vi "getNodeName.vi"(8 "error in (no error)":errorcluster, 11 "NativeXML in":refnum<class "NativeXML.lvclass">) -> (0 "error out":errorcluster, 2 "name":string, 3 "NativeXML out":refnum<class "NativeXML.lvclass">)   [LabVIEW 2011, in "Tools.lvlib" / "xml.lvlib" / "NativeXML.lvclass"]
uses:
  NativeXML.lvclass
  NativeXML.lvclass/NativeXML.ctl
  Program Files/National Instruments/LabVIEW 2011/resource/objmgr/DOMUserDefRef.rc
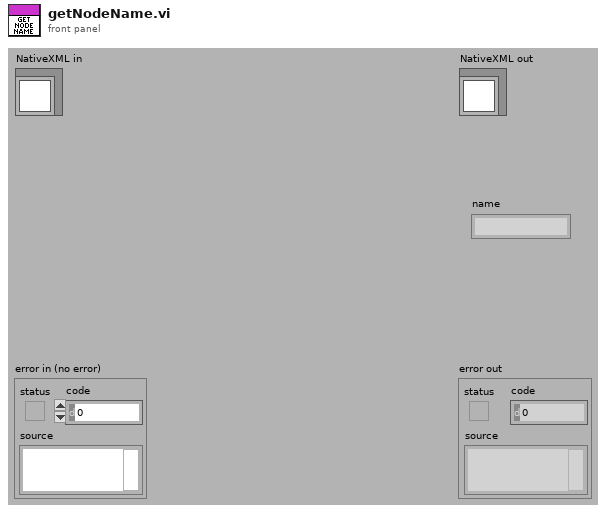
[diagram p1: front panel]
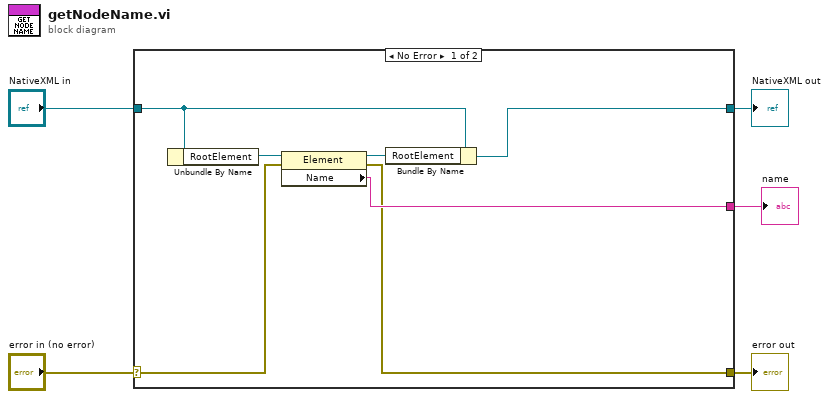
[diagram p0: block diagram]
diagram:
  n1 = case shown="No Error" "error in (no error)" {
    selector: "error in (no error)" -> [w6 w14]
    tunnel: [w7 w14] -> w4
    tunnel: [w8 w13] -> w2
    tunnel: "NativeXML in" -> [w9 w13]
    tunnel: [w11 _] -> w1
    frame No Error {
      n2 = Unbundle By Name(w9) -> ("RootElement"=w12:refnum<k20>)
      n3 = property class="Element"(reference=w12, error in=w6) -> (reference out=w10:refnum<k20>, error out=w7:errorcluster, "Name"=w11:string)
      n4 = Bundle By Name(cluster=w9, "RootElement"=w10) -> (w8:refnum<class "NativeXML.lvclass">)
    }
    frame Error {
    }
  }
  "error out" <- w4
  "NativeXML out" <- w2
  "name" <- w1
